vi "JK flip flop.vi"() -> ()   [LabVIEW 2021]
panel:
  in  "Clock":bool
  in  "K":bool
  in  "J":bool
  out "Q'":bool
  out "Q":bool
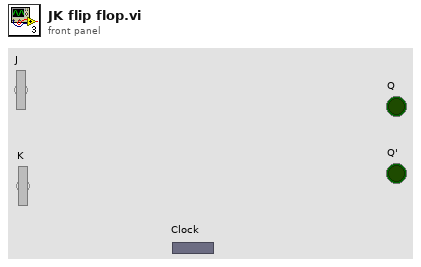
[diagram p1: front panel]
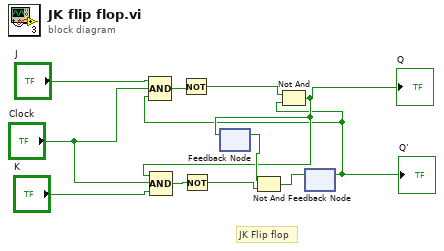
[diagram p0: block diagram]
diagram:
  # "JK Flip flop"
  n1 = feedback #1() -> (w11:bool)  [unwired: 1 in]
  n2 = feedback #2() -> (w1:bool)  [unwired: 1 in]
  "Q'" <- w1
  n3 = Compound Arithmetic op=AND("J", "Clock", w1) -> (w10:bool)
  n4 = Not(x=w10) -> (.not. x?=w8:bool)
  n5 = Not And(1:w1, 2:w8) -> (0:w3:bool)
  "Q" <- w3
  n6 = Compound Arithmetic op=AND(w3, "Clock", "K") -> (w9:bool)
  n7 = Not(x=w9) -> (.not. x?=w7:bool)
  n8 = feedback-in #1(w3) -> ()
  n9 = Not And(1:w7, 2:w11) -> (0:w2:bool)
  n10 = feedback-in #2(w2) -> ()
